vi "About Data Logger.vi"(8 "Error In":errorcluster) -> (0 "Error Out":errorcluster)   [LabVIEW 2014]
panel:
  # "Ehsan Peymani"
  # "Home Project"
  # "Data Logging Application Software"
  # "https://www.linkedin.com/in/phdingehsanpeymani/"
  # "Click in window to continue ..."
  # "© 2015 Ehsan Peymani. All rights reserved."
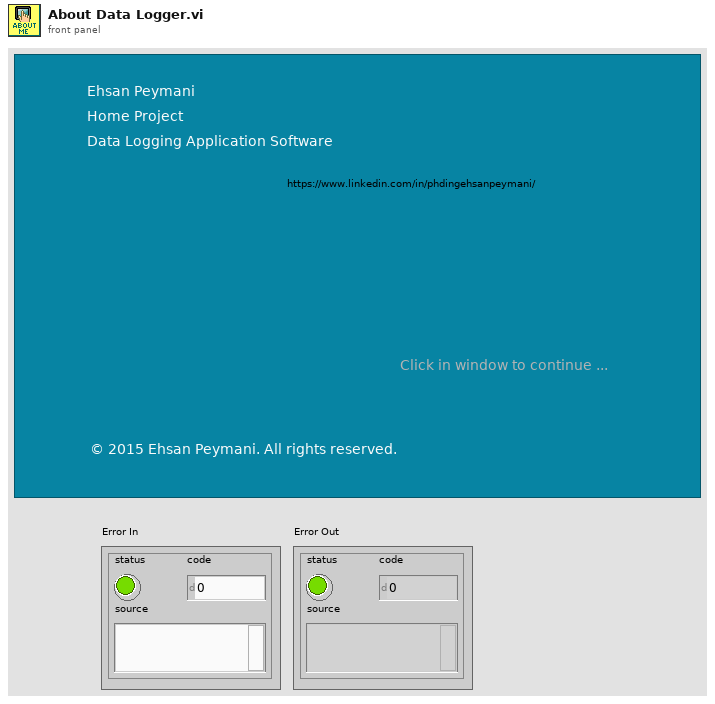
[diagram p1: front panel]
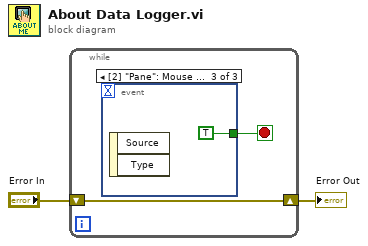
[diagram p0: block diagram]
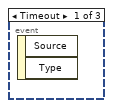
[diagram p2: hidden frame]
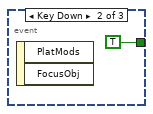
[diagram p3: hidden frame]
diagram:
  n1 = while {
    shift-right: [w3] -> w1
    shift-left: "Error In" -> [w3]
    stop <- w4 stop-if-true
    n2 = event shown="[2] \"Pane\": Mouse Down" {
      selector: _ -> [_ _ _]
      dyn-events: _ -> [_ _ _]
      timeout: _ -> [_ _ _]
      tunnel: [_ TRUE TRUE] -> w4
      event Timeout {
        n3 = event-data() -> ()  [unwired: 1 in, 2 out]
      }
      event Key Down {
        n4 = event-data() -> ()  [unwired: 1 in, 2 out]
      }
      event Mouse Down {
        n5 = event-data() -> ()  [unwired: 1 in, 2 out]
      }
    }
  }
  "Error Out" <- w1
